vi "Read Message.vi"(8 "error in":errorcluster, 11 "EF20 in":refnum<class "EF20.lvclass">) -> (0 "error out":errorcluster, 2 "Read Data":u8[](array[numeric]) format="%.0x", 3 "EF20 out":refnum<class "EF20.lvclass">)   [LabVIEW 2018, in "EF20.lvlib" / "EF20.lvclass"]
uses:
  EF20.lvclass
  PPLs/Oven/Oven.lvlibp/Oven.lvclass
  C:/Projects/LabVIEW/PPLs/Oven/Oven.lvlibp/Oven.lvclass
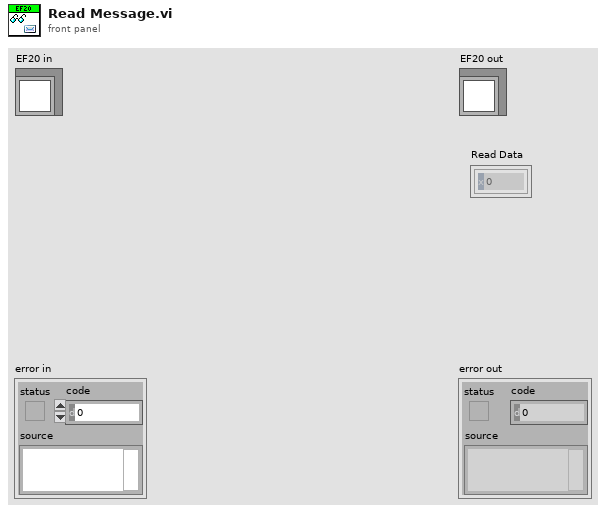
[diagram p1: front panel]
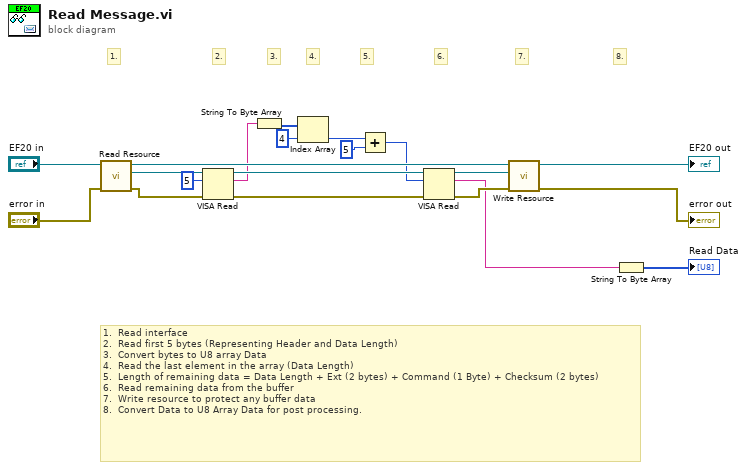
[diagram p0: block diagram]
diagram:
  # "1.  Read interface\n2.  Read first 5 bytes (Representing Header and Data Length)\n3.  Convert bytes to U8 array Data\n4.  Read the last element in the array (Data Length)\n5.  Length of remaining data = Data Length + Ext (2 bytes) + Command (1 Byte) + Checksum (2 bytes)\n6.  Read remaining data from the buffer\n7.  Write resource to protect any buffer data\n8.  Convert Data to U8 Array Data for post processing."
  # "8."
  # "7."
  # "6."
  # "5."
  # "4."
  # "3."
  # "2."
  # "1."
  n1 = call "Read Resource.vi"("error in (no error)"="error in", "Oven in"="EF20 in") -> ("error out"=w9:errorcluster, "Resource"=w19:refnum<visa-resource-name>, "Oven out"=w20:refnum<class "EF20.lvclass">)  [unwired: 7 in]
  n2 = VISA Read(VISA resource name=w19, byte count=u32 5, error in (no error)=w9) -> (VISA resource name out=w10:refnum<visa-resource-name>, read buffer=w7:string, error out=w6:errorcluster)  [unwired: 1 out]
  n3 = String To Byte Array(string=w7) -> (unsigned byte array=w5:u8[])
  n4 = Index Array(array=w5, index=4) -> (element=w3:u8)
  n5 = Add(x=w3, y=u8 5 ("x")) -> (x+y=w2:u8)
  n6 = VISA Read(VISA resource name=w10, byte count=w2, error in (no error)=w6) -> (VISA resource name out=w18:refnum<visa-resource-name>, read buffer=w12:string, error out=w14:errorcluster)  [unwired: 1 out]
  n7 = call "Write Resource.vi"("error in (no error)"=w14, "Resource"=w18, "Oven in"=w20) -> ("error out"=→"error out":errorcluster, "Oven out"=→"EF20 out":refnum<class "EF20.lvclass">)  [unwired: 7 in]
  n8 = String To Byte Array(string=w12) -> (unsigned byte array=→"Read Data":u8[])
